vi "main.vi"() -> ()   [LabVIEW 2022 SP3]
panel:
  out "TCPIP error out":errorcluster
  out "GPIB error out":errorcluster
  in  "GPIB error in":errorcluster
  in  "TCPIP error in":errorcluster
  out "Risposta Inviata al Client":string[](array[string])
  in  "ATE Control parameter":T1(array[cluster])=[{"Device"=10, "Operation"=0, "Command/byte count"="OUTP:LOAD INF\nAPPL:SIN 1000,10,0"}, {"Device"=1, "Operation"=0, "Command/byte count"="HEAD OFF\nDAT:SOU CH1\nDAT:ENC ASCI\nDAT:WID 1\nDAT:STAR 1\nDAT:STOP 2500\nCH1:SCA 1\nHOR:MAI:SCA 250E-6\nCURV?"}, {"Device"=1, "Operation"=1, "Command/byte count"="15000"}] {"Operation" items=["write", "read"]; "Device" items=["DSO"=1, "AWG"=10]}
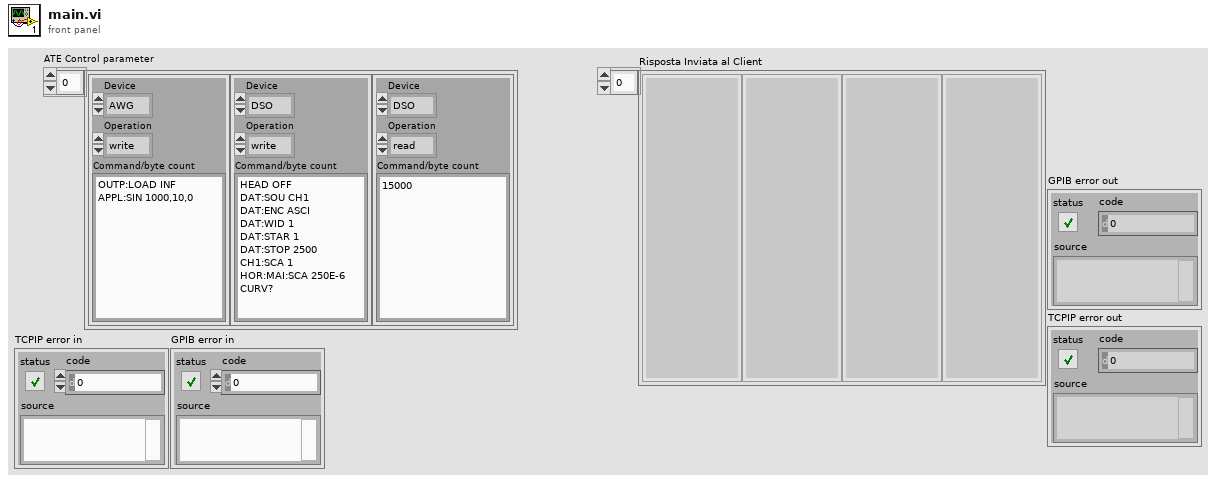
[diagram p1: front panel]
types:
  T1 = cluster{"Device":u16, "Operation":u16, "Command/byte count":string}[]
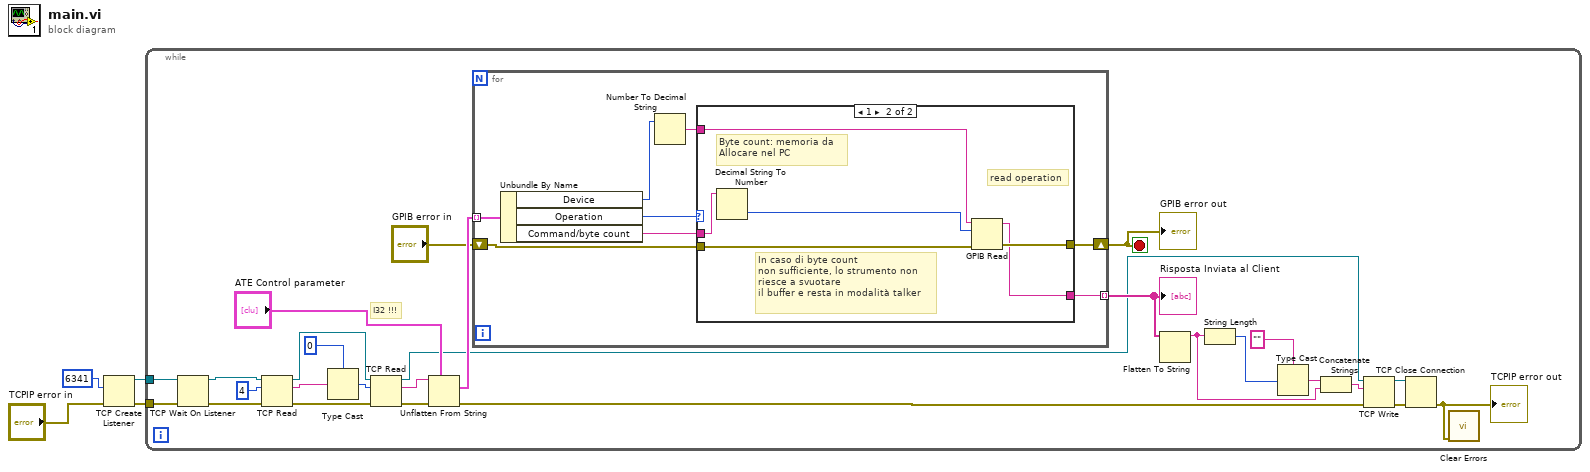
[diagram p0: block diagram]
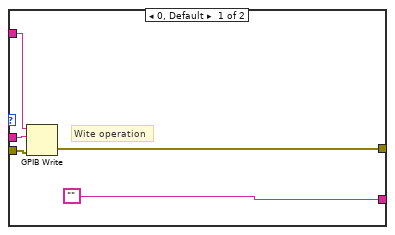
[diagram p2: hidden frame]
diagram:
  n1 = TCP Create Listener(8:"TCPIP error in", 10:u16 6341 ("port")) -> (0:w1:errorcluster, 3:w2:refnum<k5>)  [unwired: 3 in, 1 out]
  n2 = while {
    tunnel: w2 -> [w31]
    tunnel: w1 -> [w5]
    stop <- w17 stop-if-true
    # "I32 !!!"
    n3 = TCP Wait On Listener(8:w5, 11:w31) -> (0:w29:errorcluster, 3:w30:refnum<k5>)  [unwired: 2 in, 3 out]
    n4 = TCP Read(connection ID=w30, bytes to read=4, error in (no error)=w29) -> (connection ID out=w24:refnum<k5>, data out=w27:string, error out=w23:errorcluster)  [unwired: 2 in]
    n5 = Type Cast(type=0, x=w27) -> (*(type *) &x=w25:i32)
    n6 = TCP Read(connection ID=w24, bytes to read=w25, error in (no error)=w23) -> (connection ID out=w12:refnum<k5>, data out=w22:string, error out=w21:errorcluster)  [unwired: 2 in]
    n7 = Unflatten From String(type="ATE Control parameter", binary string=w22, error in (no error)=w21) -> (value=w19:T1, error out=w10:errorcluster)  [unwired: 2 in, 1 out]
    n8 = for {
      tunnel: w19 -> [w39] mode=indexing
      shift-right: [w33] -> w17
      shift-left: "GPIB error in" -> [w34]
      tunnel: [w32] -> w18 mode=indexing
      n9 = Unbundle By Name(w39) -> ("Device"=w38:u16, "Operation"=w37:u16, "Command/byte count"=w35:string)
      n10 = Number To Decimal String(number=w38) -> (decimal integer string=w36:string)  [unwired: 1 in]
      n11 = case shown="1" w37 {
        tunnel: w36 -> [w44 w49]
        tunnel: w35 -> [w43 w48]
        tunnel: w34 -> [w42 w50]
        tunnel: [w41 w46] -> w33
        tunnel: ["" w45] -> w32
        frame 0, Default {
          # "Wite operation"
          n12 = GPIB Write(0:w44, 1:w43, 3:w42) -> (6:w41:errorcluster)  [unwired: 2 in, 1 out]
        }
        frame 1 {
          # "In caso di byte count\nnon sufficiente, lo strumento non\nriesce a svuotare\nil buffer e resta in modalità talker"
          # "Byte count: memoria da\nAllocare nel PC"
          # "read operation"
          n13 = Decimal String To Number(string=w48) -> (number=w47:i32)  [unwired: 2 in, 1 out]
          n14 = GPIB Read(0:w49, 1:w47, 3:w50) -> (5:w45:string, 7:w46:errorcluster)  [unwired: 2 in, 1 out]
        }
      }
    }
    "Risposta Inviata al Client" <- w18
    "GPIB error out" <- w17
    n15 = Flatten To String(anything=w18) -> (data string=w13:string)  [unwired: 3 in, 2 out]
    n16 = String Length(string=w13) -> (length=w16:i32)
    n17 = Type Cast(type="", x=w16) -> (*(type *) &x=w14:string)
    n18 = Concatenate Strings(w14, w13) -> (w11:string)
    n19 = TCP Write(connection ID=w12, data in=w11, error in (no error)=w10) -> (connection ID out=w7:refnum<k5>, error out=w8:errorcluster)  [unwired: 1 in, 1 out]
    n20 = TCP Close Connection(connection ID=w7, error in (no error)=w8) -> (error out=w6:errorcluster)  [unwired: 1 in, 1 out]
    "TCPIP error out" <- w6
    n21 = call <vilib>:"Clear Errors.vi"("error in (no error)"=w6) -> ()  [unwired: 5 in, 2 out]
  }
